vi "Write Scale.vi"(8 "error in (no error)":errorcluster, 10 "Scale":dbl, 11 "Parameter in":refnum<class "Parameter.lvclass">) -> (0 "error out":errorcluster, 3 "Parameter out":refnum<class "Parameter.lvclass">)   [LabVIEW 2013, in "Parameter.lvclass"]
uses:
  Parameter.lvclass
  Parameter.lvclass/Parameter.ctl
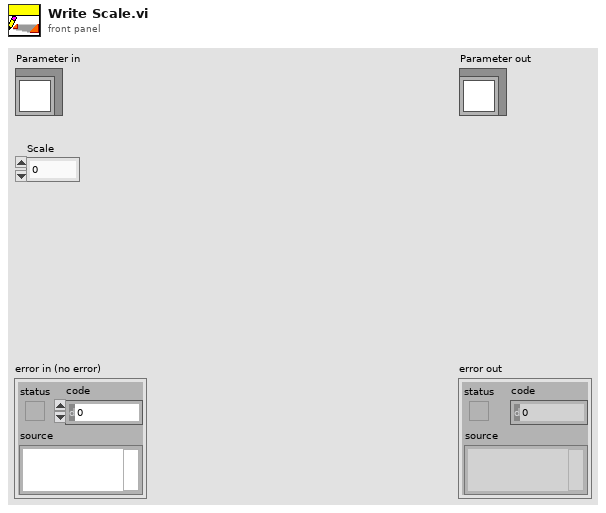
[diagram p1: front panel]
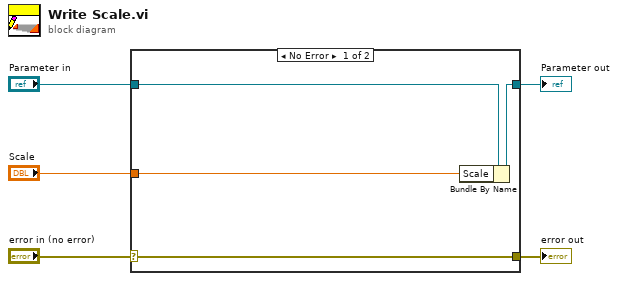
[diagram p0: block diagram]
diagram:
  n1 = case shown="No Error" "error in (no error)" {
    selector: "error in (no error)" -> [w9 w10]
    tunnel: [w9 w10] -> w4
    tunnel: [w7 w11] -> w2
    tunnel: "Parameter in" -> [w8 w11]
    tunnel: "Scale" -> [w6 _]
    frame No Error {
      n2 = Bundle By Name(cluster=w8, "Scale"=w6) -> (w7:refnum<class "Parameter.lvclass">)
    }
    frame Error {
    }
  }
  "error out" <- w4
  "Parameter out" <- w2
